vi "Test Add and Undo All.vi"(8 "error in":errorcluster, 11 "Test Case In":refnum<class "History Tests.lvclass">) -> (0 "error out":errorcluster, 3 "Test Case Out":refnum<class "History Tests.lvclass">)   [LabVIEW 2020, in "History Tests.lvclass"]
doc: "Adds many states to the undo buffer and then performs an Undo on all of the added states."
uses:
  History Tests.lvclass
  History Tests.lvclass/History Tests.ctl
  C:/Program Files/National Instruments/LabVIEW 2026/vi.lib/Astemes/LUnit/Test Case.lvclass
  C:/Program Files/National Instruments/LabVIEW 2026/vi.lib/Astemes/LUnit/LUnit Runnable.lvclass
  C:/Users/J63553/Projects/_LabVIEW Community/labview-icon-editor/Test/Unit Tests/History Tests/History Tests.lvclass
  resource/plugins/NIIconEditor/History/History/History.lvclass
  <vilib>/Astemes/LUnit/Test Case.lvclass
panel:
  out "Have Changes":bool
  out "Undo Data":string[](array[string])
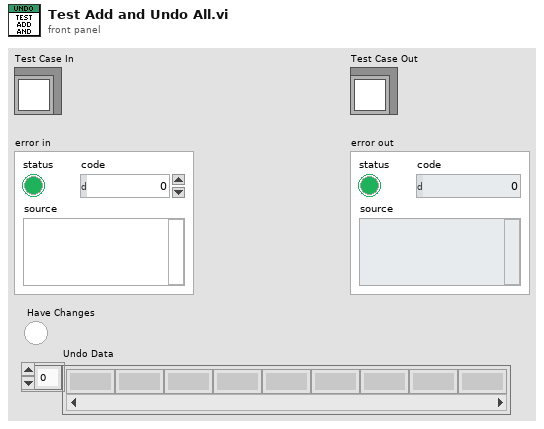
[diagram p1: front panel]
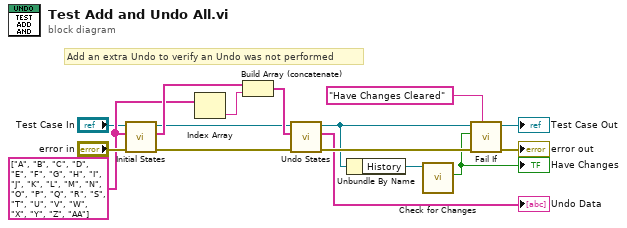
[diagram p0: block diagram]
diagram:
  w11 = string[] ["A", "B", "C", "D", "E", "F", "G", "H", "I", "J", "K", "L", "M", "N", "O", "P", "Q", "R", "S", "T", "U", "V", "W", "X", "Y", "Z", "AA"]
  # "Add an extra Undo to verify an Undo was not performed"
  n1 = call "Initial States.vi"("error in"="error in", "States"=w11, "Test Case In"="Test Case In") -> ("error out"=w15:errorcluster, "Expected Undo Stack"=w12:string[], "Test Case Out"=w7:refnum<class "History Tests.lvclass">)  [unwired: 5 in, 1 out]
  n2 = Index Array(array=w11) -> (element=w10:string)  [unwired: 1 in]
  n3 = Build Array (concatenate)(w12, w10) -> (w9:string[])
  n4 = call "Undo States.vi"("error in"=w15, "Expected Undo States"=w9, "Test Case In"=w7) -> ("error out"=w14:errorcluster, "Actual Undo States"=→"Undo Data":string[], "Test Case Out"=w2:refnum<class "History Tests.lvclass">)  [unwired: 6 in]
  n5 = Unbundle By Name(w2) -> ("History"=w5:refnum<class "History.lvclass">)
  n6 = call "Check for Changes.vi"("History"=w5) -> ("Have Changes"=w1:bool)  [unwired: 10 in]
  "Have Changes" <- w1
  n7 = call <vilib>:"Fail If.vi"("Description"="Have Changes Cleared", "error in (no error)"=w14, "Fail?"=w1, "LUnit Test Case In"=w2) -> ("error out"=→"error out":errorcluster, "LUnit Test Case Out"=→"Test Case Out":refnum<class "History Tests.lvclass">)  [unwired: 6 in]
